vi "[Generate Test Cases] Fix path.vi"() -> (3 "Fix Path test cases":refnum<class "TestCase.lvclass">[](array[class]))   [LabVIEW 2015, in "Tests.lvlib" / "[Test Suite] File Transfer Helpers.lvclass"]
uses:
  [Test Suite] File Transfer Helpers.lvclass
  <vilib>/addons/_JKI Toolkits/VI Tester/TestCase.llb/TestCase.lvclass
  [Test Case] Fix Path/[Test Case] Fix path.lvclass
  [Test Case] Fix Path/[Test Case] Fix path.lvclass/[Test Case] Fix path.ctl
  [Test Case] Fix Path/Write Path in.vi
  [Test Case] Fix Path/Write Expected path out.vi
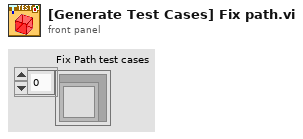
[diagram p1: front panel]
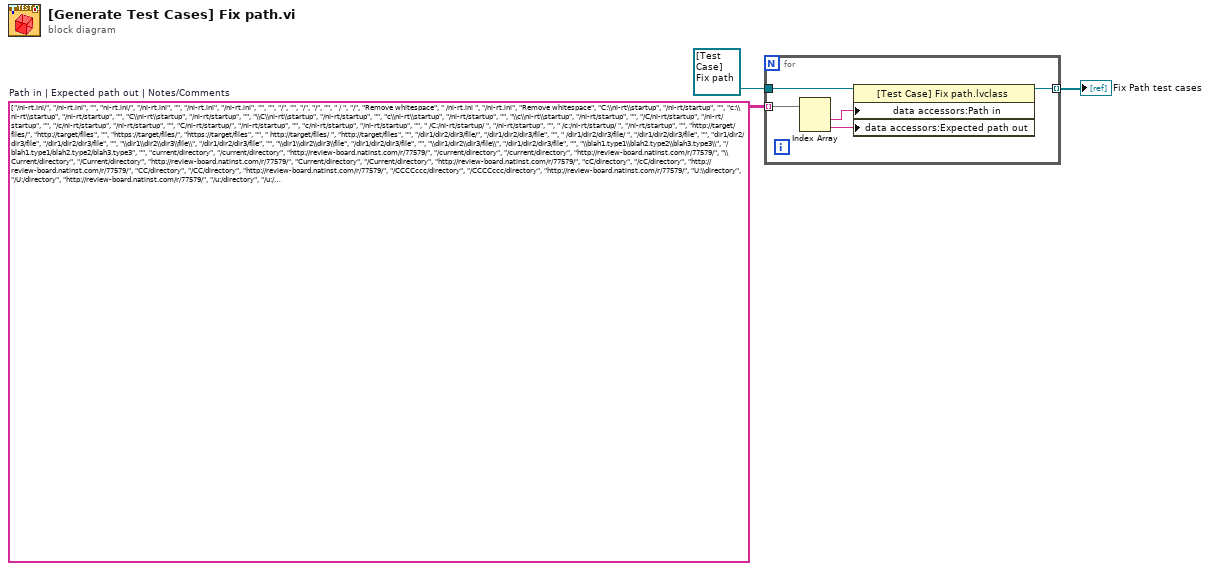
[diagram p0: block diagram]
diagram:
  w1 = string[][] [["/ni-rt.ini/", "/ni-rt.ini", ""], ["ni-rt.ini/", "/ni-rt.ini", ""], ["/ni-rt.ini", "/ni-rt.ini", ""], ["", "/", ""], ["/", "/", ""], [" / ", "/", "Remove whitespace"], [" /ni-rt.ini ", "/ni-rt.ini", "Remove whitespace"], ["C:\\ni-rt\\startup", "/ni-rt/startup", ""], ["c:\\ni-rt\\startup", "/ni-rt/startup", ""], ["C\\ni-rt\\startup", "/ni-rt/startup", ""], ["\\C\\ni-rt\\startup", "/ni-rt/startup", ""], ["c\\ni-rt\\startup", "/ni-rt/startup", ""], ["\\c\\ni-rt\\startup", "/ni-rt/startup", ""], ["/C/ni-rt/startup", "/ni-rt/startup", ""], ["/c/ni-rt/startup", "/ni-rt/startup", ""], ["C/ni-rt/startup/", "/ni-rt/startup", ""], ["c/ni-rt/startup", "/ni-rt/startup", ""], [" /C:/ni-rt/startup/ ", "/ni-rt/startup", ""], [" /c:/ni-rt/startup/ ", "/ni-rt/startup", ""], ["http://target/files/", "http://target/files", ""], ["https://target/files/", "https://target/files", ""], [" http://target/files/ ", "http://target/files", ""], ["/dir1/dir2/dir3/file/", "/dir1/dir2/dir3/file", ""], [" /dir1/dir2/dir3/file/ ", "/dir1/dir2/dir3/file", ""], ["dir1/dir2/dir3/file", "/dir1/dir2/dir3/file", ""], ["\\dir1\\dir2\\dir3\\file\\", "/dir1/dir2/dir3/file", ""], ["\\dir1\\dir2\\dir3\\file", "/dir1/dir2/dir3/file", ""], ["\\dir1/dir2\\dir3/file\\", "/dir1/dir2/dir3/file", ""], ["\\blah1.type1\\blah2.type2\\blah3.type3\\", "/blah1.type1/blah2.type2/blah3.type3", ""], ["current/directory", "/current/directory", "http://review-board.natinst.com/r/77579/"], ["/current/directory", "/current/directory", "http://review-board.natinst.com/r/77579/"], ["\\Current/directory", "/Current/directory", "http://review-board.natinst.com/r/77579/"], ["Current/directory", "/Current/directory", "http://review-board.natinst.com/r/77579/"], ["cC/directory", "/cC/directory", "http://review-board.natinst.com/r/77579/"], ["CC/directory", "/CC/directory", "http://review-board.natinst.com/r/77579/"], ["/CCCCccc/directory", "/CCCCccc/directory", "http://review-board.natinst.com/r/77579/"], ["U:\\directory", "/U:/directory", "http://review-board.natinst.com/r/77579/"], ["/u:/directory", "/u:/directory", "http://review-board.natinst.com/r/77579/"], ["\\w:/directory", "/w:/directory", "http://review-board.natinst.com/r/77579/"], ["/w/directory", "/w/directory", "http://review-board.natinst.com/r/77579/"]]  # Path in | Expected path out | Notes/Comments
  n1 = for {
    tunnel: refnum<class "[Test Case] Fix path.lvclass"> refnum ("[Test Case] Fix Path.lvclass") -> [w8]
    tunnel: [w7] -> w2 mode=indexing
    tunnel: w1 -> [w6] mode=indexing
    n2 = Index Array(array=w6) -> (element #1=w5:string, element #2=w4:string)  [unwired: 2 in]
    n3 = property class="[Test Case] Fix path.lvclass"(reference=w8, "data accessors:Path in"=w5, "data accessors:Expected path out"=w4) -> (reference out=w7:refnum<class "[Test Case] Fix path.lvclass">)  [unwired: 1 in, 1 out]
  }
  "Fix Path test cases" <- w2
